vi "Work Position.vi"(8 "Work position parameter":i32[](array[numeric]), 9 "Noise":dbl[](array[numeric]), 10 "A\\B":dbl[](array[numeric]), 11 "S":dbl[](array[numeric])) -> (0 "A\\B_2nd_part":dbl[](array[numeric]), 1 "S_2nd_part":dbl[](array[numeric]), 2 "A\\B_1st_part":dbl[](array[numeric]), 3 "S_1st_part":dbl[](array[numeric]), 4 "Noise_2nd_part":dbl[](array[numeric]), 5 "Noise_1st_part":dbl[](array[numeric]))   [LabVIEW 2015, in "Digital Signal Processing.lvlib"]
uses:
  Digital Signal Processing.lvlib
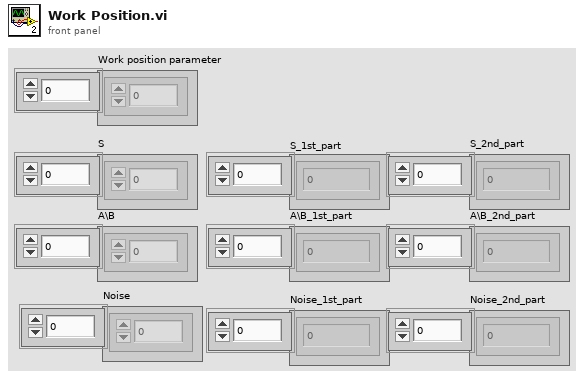
[diagram p1: front panel]
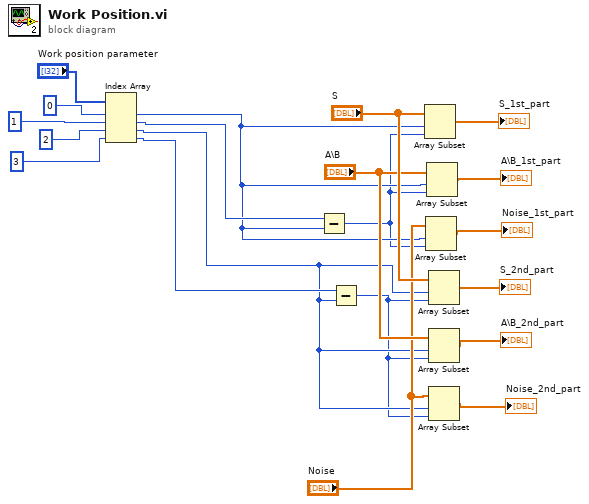
[diagram p0: block diagram]
diagram:
  n1 = Index Array(array="Work position parameter", index #1=0 ("索引"), index #2=1 ("索引"), index #3=2 ("索引"), index #4=3 ("索引")) -> (element #1=w6:i32, element #2=w9:i32, element #3=w4:i32, element #4=w8:i32)
  n2 = Subtract(x=w9, y=w6) -> (x-y=w5:i32)
  n3 = Subtract(x=w8, y=w4) -> (x-y=w3:i32)
  n4 = Array Subset(array="S", index=w6, length=w5) -> (→"S_1st_part":dbl[])
  n5 = Array Subset(array="Noise", index=w6, length=w5) -> (→"Noise_1st_part":dbl[])
  n6 = Array Subset(array="A\\B", index=w6, length=w5) -> (→"A\\B_1st_part":dbl[])
  n7 = Array Subset(array="S", index=w4, length=w3) -> (→"S_2nd_part":dbl[])
  n8 = Array Subset(array="A\\B", index=w4, length=w3) -> (→"A\\B_2nd_part":dbl[])
  n9 = Array Subset(array="Noise", index=w4, length=w3) -> (→"Noise_2nd_part":dbl[])
